vi "Update Plugin UI Tab Name.vi"(8 "error in (no error)":errorcluster, 10 "Plugin Name":string, 11 "CIF_UI in":refnum<class "CIF_UI.lvclass">) -> (0 "error out":errorcluster)   [LabVIEW 2021, in "CIF_UI.lvclass"]
uses:
  CIF_UI.lvclass
  CIF_UI.lvclass/CIF_UI.ctl
  Typedef/CIF_Manager_UI_Tab.ctl
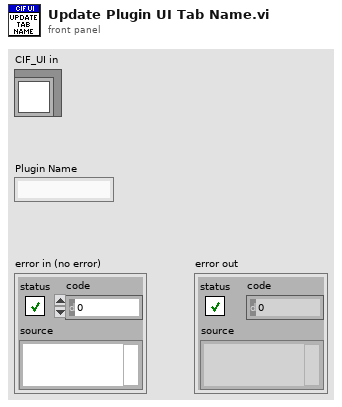
[diagram p1: front panel]
types:
  T1 = typedef "CIF_Manager_UI_Tab.ctl" = enum32{"System Management", "Channels", "Monitoring and Errors", "Plugin UI"}
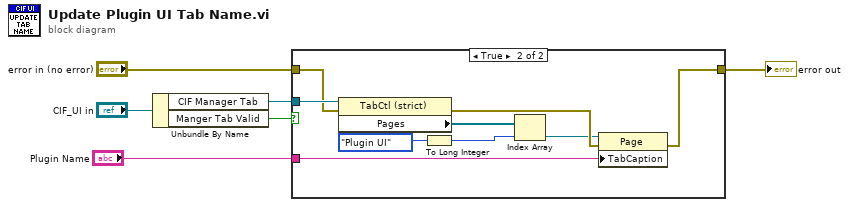
[diagram p0: block diagram]
diagram:
  n1 = Unbundle By Name("CIF_UI in") -> ("CIF Manager Tab"=w4:refnum<vi>, "Manger Tab Valid"=w5:bool)
  n2 = case shown="True" w5 {
    tunnel: w4 -> [_ w16]
    tunnel: "error in (no error)" -> [w7 w14]
    tunnel: [w7 w13] -> w2
    tunnel: "Plugin Name" -> [_ w8]
    frame False {
    }
    frame True {
      n3 = property class="TabCtl (strict)"(reference=w16, error in=w14) -> (error out=w15:errorcluster, "Pages"=w12:refnum<vi>[])  [unwired: 1 out]
      n4 = To Long Integer(number=CIF_Manager_UI_Tab."Plugin UI" ("y")) -> (32bit integer=w10:i32)
      n5 = Index Array(array=w12, index=w10) -> (element=w9:refnum<vi>)
      n6 = property class="Page"(reference=w9, error in=w15, "TabCaption"=w8) -> (error out=w13:errorcluster)  [unwired: 1 out]
    }
  }
  "error out" <- w2
